vi "20150719_Online_Program_emergency.vi"() -> ()   [LabVIEW 2014]
uses:
  <vilib>/Utility/file.llb/Read From Spreadsheet File (DBL).vi
  <vilib>/Analysis/Matrix/Numeric/Conversions/Array To Matrix - RA2.vi
  <vilib>/Analysis/Matrix/Numeric/Conversions/Array To Matrix - RA.vi
  <vilib>/Utility/file.llb/Write To Spreadsheet File (DBL).vi
  <vilib>/Utility/file.llb/Write To Spreadsheet File (I64).vi
  <vilib>/Analysis/Matrix/NI_Matrix.lvlib
  <vilib>/Instr/_visa.llb/VISA Configure Serial Port (Instr).vi
  NeuroSky_Dll_Call/Debug/NeuroSky_Dll_Call.dll
  user32.dll
panel:
  out "에러 출력":errorcluster
  out "메시지 2":string
  out "큐사인":bool
  out "icon_온도":bool
  out "icon_용변":bool
  out "icon_자판":bool
  out "icon_응급":bool=TRUE
  out "icon_기계":bool
  out "icon_침대":bool
  out "메시지":string
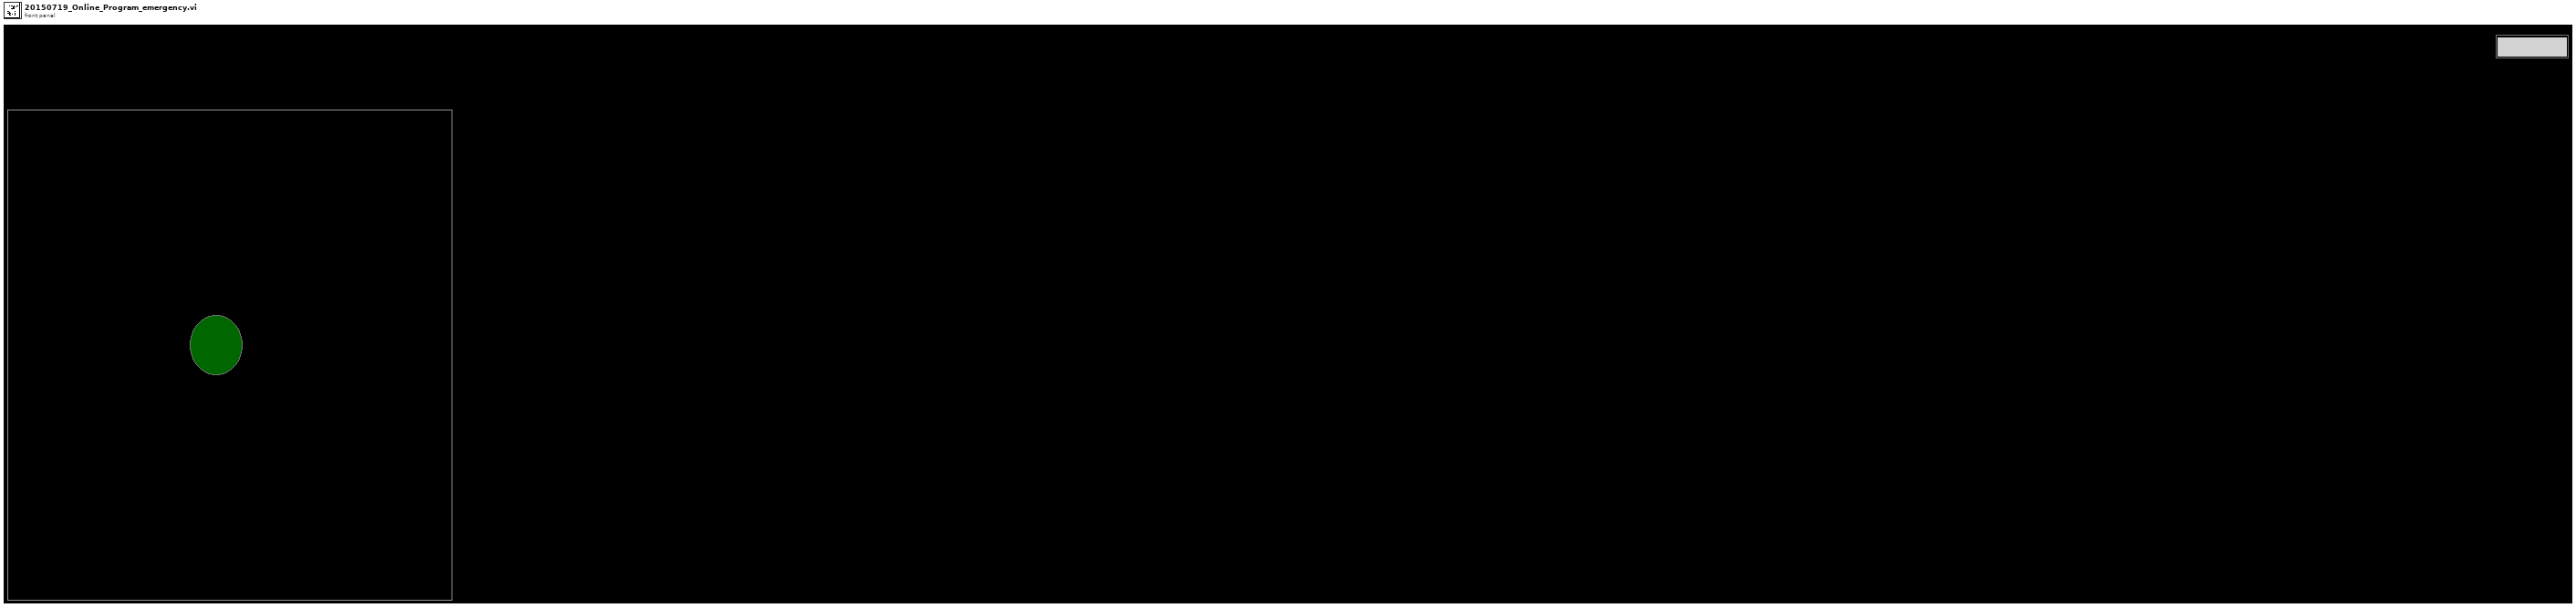
[diagram p1: front panel]
types:
  T1 = typedef "NI_Matrix.lvlib/RealMatrix.ctl" = dbl[][]
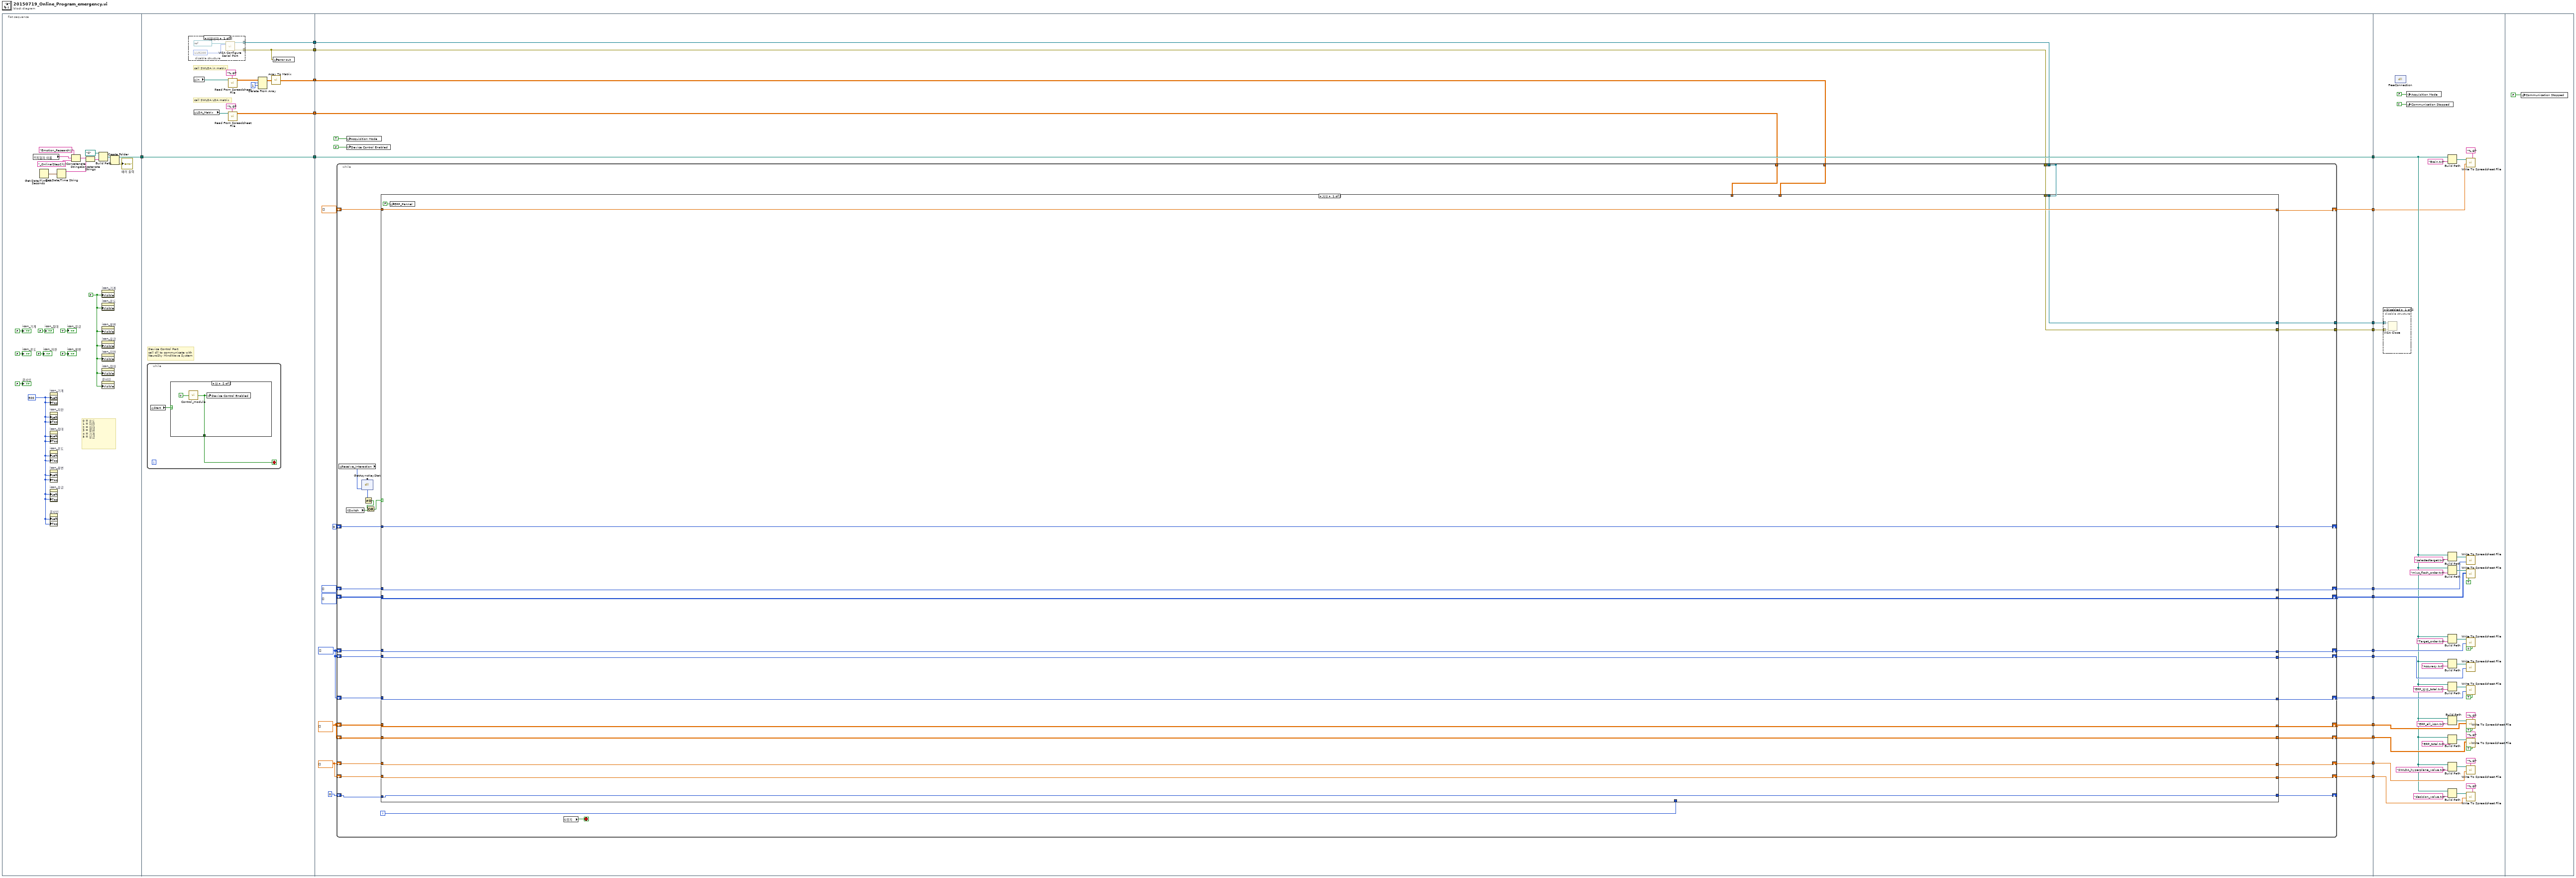
[diagram p0: block diagram]
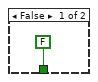
[diagram p3: hidden frame]
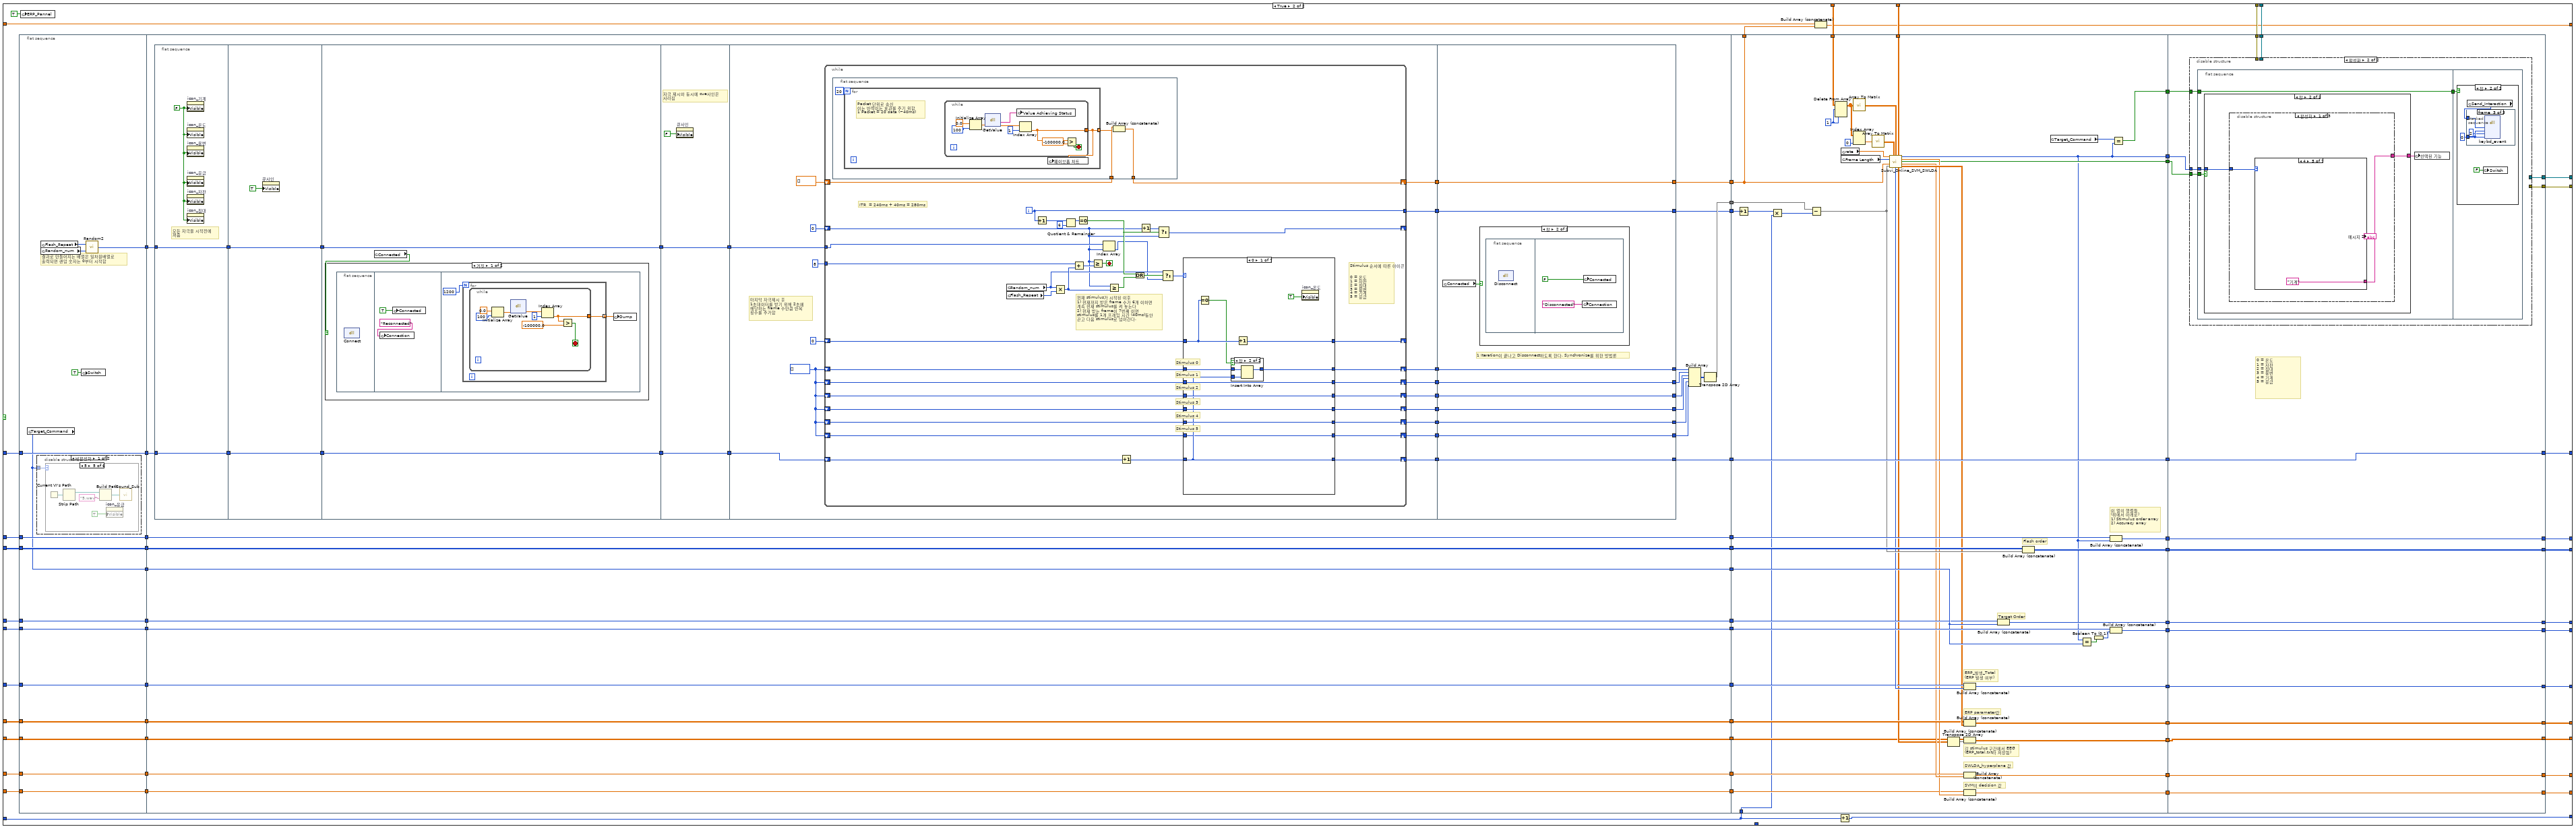
[diagram p4: hidden frame]
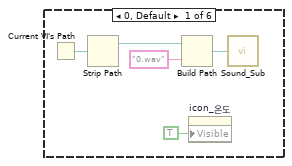
[diagram p5: hidden frame]
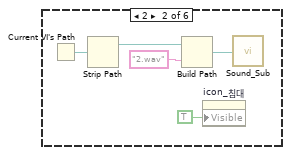
[diagram p6: hidden frame]
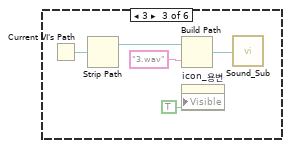
[diagram p7: hidden frame]
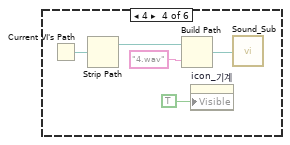
[diagram p8: hidden frame]
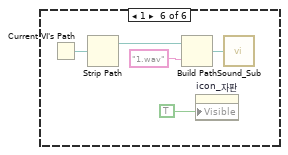
[diagram p9: hidden frame]
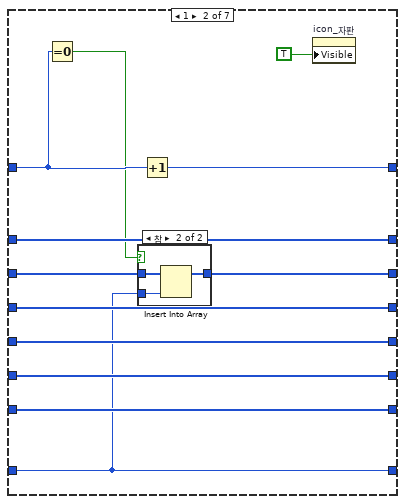
[diagram p13: hidden frame]
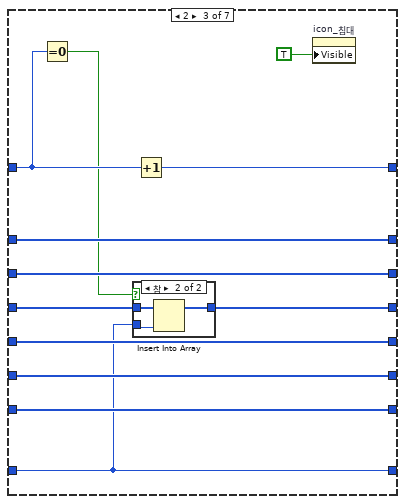
[diagram p15: hidden frame]
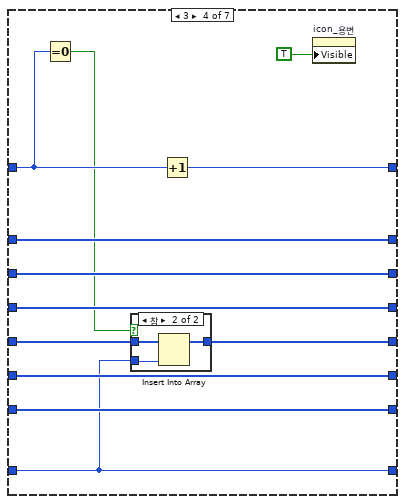
[diagram p17: hidden frame]
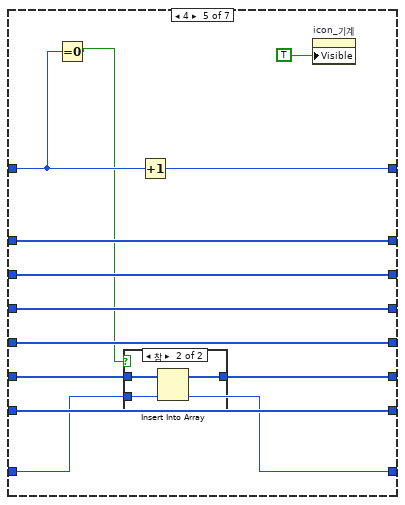
[diagram p19: hidden frame]
diagram:
  n1 = flat-sequence {
    tunnel: [w39] -> w19
    tunnel: w19 -> [w51]
    tunnel: [w51] -> w18
    tunnel: [w49] -> w17
    tunnel: [w42] -> w7
    tunnel: [w41] -> w4
    tunnel: [w40] -> w3
    tunnel: w18 -> [w78]
    tunnel: [w78] -> w16
    tunnel: [w87] -> w15
    tunnel: [w85] -> w14
    tunnel: [w83] -> w13
    tunnel: w17 -> [w68]
    tunnel: [w82] -> w12
    tunnel: [w79] -> w11
    tunnel: [w75] -> w10
    tunnel: [w74] -> w9
    tunnel: [w73] -> w8
    tunnel: w7 -> [w67]
    tunnel: [w71] -> w6
    tunnel: [w69] -> w5
    tunnel: w4 -> [w66]
    tunnel: w3 -> [w65]
    tunnel: [w64] -> w2
    tunnel: [w63] -> w1
    tunnel: w16 -> [w725]
    tunnel: w15 -> [w720]
    tunnel: w14 -> [w759]
    tunnel: w13 -> [w755]
    tunnel: w12 -> [w752]
    tunnel: w11 -> [w748]
    tunnel: w10 -> [w742]
    tunnel: w9 -> [w737]
    tunnel: w8 -> [w734]
    tunnel: w6 -> [w731]
    tunnel: w5 -> [w726]
    tunnel: w2 -> [w722]
    tunnel: w1 -> [w721]
    frame #0 {
      w21 = FALSE ("Visible")
      w22 = 500 ("Position:Left")
      # "0 = 온도\n1 = 자판\n2 = 침대\n3 = 용변 \n4 = 기계 \n5 = 응급"
      n2 = global read "Control_Panel_정리.vi" "피험자 이름"() -> (w30:string)
      n3 = Get Date/Time In Seconds() -> (seconds since 1Jan1904=w36:timestamp)
      n4 = property on="icon_기계" class="Bool (엄격한)"("Left"=w22, "Top"=w22) -> ()  [unwired: 2 in, 2 out]
      n5 = property on="icon_자판" class="Bool (엄격한)"("Left"=w22, "Top"=w22) -> ()  [unwired: 2 in, 2 out]
      n6 = property on="icon_침대" class="Bool (엄격한)"("Left"=w22, "Top"=w22) -> ()  [unwired: 2 in, 2 out]
      n7 = property on="icon_온도" class="Bool (엄격한)"("Left"=w22, "Top"=w22) -> ()  [unwired: 2 in, 2 out]
      n8 = property on="icon_용변" class="Bool (엄격한)"("Left"=w22, "Top"=w22) -> ()  [unwired: 2 in, 2 out]
      n9 = property on="icon_응급" class="Bool (엄격한)"("Left"=w22, "Top"=w22) -> ()  [unwired: 2 in, 2 out]
      n10 = property on="큐사인" class="Bool (엄격한)"("Left"=w22, "Top"=w22) -> ()  [unwired: 2 in, 2 out]
      n11 = Get Date/Time String(seconds (now)=w36) -> (date string=w37:string)  [unwired: 2 in, 1 out]
      n12 = Concatenate Strings("Emotion_Research\\" ("string"), w30, "_Online(Step2)\\" ("문자열")) -> (w32:string)
      n13 = Concatenate Strings(w32, w37) -> (w34:string)
      n14 = Build Path(base path=path "C:/" ("path"), name or relative path=w34) -> (appended path=w35:path)
      n15 = property on="icon_기계" class="Bool (엄격한)"("Visible"=w21) -> ()  [unwired: 2 in, 2 out]
      n16 = property on="icon_온도" class="Bool (엄격한)"("Visible"=w21) -> ()  [unwired: 2 in, 2 out]
      n17 = property on="icon_용변" class="Bool (엄격한)"("Visible"=w21) -> ()  [unwired: 2 in, 2 out]
      n18 = property on="icon_응급" class="Bool (엄격한)"("Visible"=w21) -> ()  [unwired: 2 in, 2 out]
      n19 = property on="icon_자판" class="Bool (엄격한)"("Visible"=w21) -> ()  [unwired: 2 in, 2 out]
      n20 = property on="icon_침대" class="Bool (엄격한)"("Visible"=w21) -> ()  [unwired: 2 in, 2 out]
      n21 = property on="큐사인" class="Bool (엄격한)"("Visible"=w21) -> ()  [unwired: 2 in, 2 out]
      n22 = Create Folder(path (use dialog)=w35) -> (created path=w39:path, error out=→"에러 출력":errorcluster)  [unwired: 2 in, 1 out]
      "icon_온도" <- FALSE ("icon_전원 6")
      "icon_용변" <- FALSE ("icon_전체종료")
      "icon_자판" <- FALSE ("icon_음량업 2")
      "icon_응급" <- TRUE ("icon_채널다운")
      "icon_기계" <- FALSE ("icon_음량다")
      "icon_침대" <- FALSE ("icon_채널업")
      "큐사인" <- FALSE ("icon_전원 7")
    }
    frame #1 {
      w45 = 1 ("인덱스 (행)")
      # "call SWLDA in matrix"
      # "call SWLDA LDA matrix"
      # "Device Control Part\ncall dll to communicate with\nNeuroSky MindWave System"
      n23 = while {
        stop <- w57 stop-if-true
        n24 = global read "Control_Panel_정리.vi" "Start"() -> (w56:bool)
        n25 = case shown="참" w56 {
          tunnel: [FALSE ("Connected") w59] -> w57
          frame False {
          }
          frame True {
            n26 = call "Control_module.vi"("Turn on"=TRUE ("Device Control Enabled")) -> ("Connected"=w59:bool)
            n27 = global write "Control_Panel_정리.vi" "Device Control Enabled"(w59) -> ()
          }
        }
      }
      n28 = disable-structure shown="비활성화" {
        disable-tunnel: [w55 _] -> w41
        disable-tunnel: [w54 _] -> w40
        frame Disabled {
          n29 = call-poly "VISA Configure Serial Port"("VISA resource name"=refnum<visa-resource-name> "COM3", "baud rate (9600)"=u32 115200) -> ("VISA resource name out"=w55:refnum<visa-resource-name>, "error out"=w54:errorcluster)  [unwired: 12 in]
        }
        frame Enabled {
        }
      }
      n30 = global read "Control_Panel_정리.vi" "in"() -> (w43:path)
      n31 = global read "Control_Panel_정리.vi" "LDA_Matrix"() -> (w48:path)
      n32 = call-poly <vilib>:"Read From Spreadsheet File.vi"("format (%.3f)"="%.6f", "file path (dialog if empty)"=w43) -> ("all rows"=w44:dbl[][])  [unwired: 5 in, 4 out]
      n33 = call-poly <vilib>:"Read From Spreadsheet File.vi"("format (%.3f)"="%.6f", "file path (dialog if empty)"=w48) -> ("all rows"=w49:dbl[][])  [unwired: 5 in, 4 out]
      n34 = Delete From Array(array=w44, length=w45, index (row)=w45) -> (array with subset deleted=w46:dbl[][])  [unwired: 1 in, 1 out]
      n35 = call-poly <vilib>:"Array To Matrix.vi"("Real 2D Array"=w46) -> ("Real Matrix"=w42:T1)
      n36 = global write "Control_Panel_정리.vi" "error out"(w40) -> ()
    }
    frame #2 {
      w72 = dbl[] []
      w70 = dbl[][] []
      w62 = i16[] []
      n37 = while {
        shift-right: [w96] -> w87
        shift-left: dbl[] [] -> [w102]
        shift-right: [w123] -> _
        shift-left: 0 ("y") -> [w124]
        shift-right: [w117] -> w85
        shift-left: i32[][] [] -> [w118]
        shift-right: [w121] -> w83
        shift-left: i32[] [] -> [w122]
        shift-right: [w119] -> w82
        shift-left: w62 -> [w120]
        shift-right: [w114] -> w79
        shift-left: w62 -> [w115]
        shift-right: [w113] -> w75
        shift-left: w62 -> [w112]
        shift-right: [w111] -> w74
        shift-left: w70 -> [w110]
        shift-right: [w109] -> w73
        shift-left: w72 -> [w108]
        shift-right: [w107] -> w71
        shift-left: w72 -> [w106]
        shift-right: [w105] -> w69
        shift-left: w70 -> [w104]
        tunnel: w68 -> [w103]
        tunnel: w67 -> [w101]
        tunnel: [w99] -> _
        tunnel: w66 -> [w99]
        tunnel: w65 -> [w100]
        tunnel: [w98] -> w64
        tunnel: [w97] -> w63
        shift-right: [w88] -> _
        shift-left: 0 -> [w89]
        i -> [w116]
        stop <- w95 stop-if-true
        n38 = global read "Control_Panel_정리.vi" "Receive_Interaction"() -> (w93:u8)
        n39 = global read "Control_Panel_정리.vi" "Switch"() -> (w91:bool)
        n40 = dll-call lib="User32.dll" fn="GetAsyncKeyState"("vKey"=w93) -> ("return type"=w94:i64)  [unwired: 4 in, 2 out]
        n41 = Not Equal To 0?(x=w94) -> (x != 0?=w92:bool)
        n42 = Or(x=w92, y=w91) -> (x .or. y?=w90:bool)
        n43 = case shown="거짓" w90 {
          tunnel: w124 -> [w136 w173]
          tunnel: [w136 w172] -> w123
          tunnel: w122 -> [w135 w171]
          tunnel: [w135 w170] -> w121
          tunnel: w120 -> [w132 w169]
          tunnel: [w132 w168] -> w119
          tunnel: w118 -> [w134 w167]
          tunnel: [w134 w166] -> w117
          tunnel: w116 -> [_ _]
          tunnel: w115 -> [w133 w165]
          tunnel: [w133 w164] -> w114
          tunnel: [w131 w163] -> w113
          tunnel: w112 -> [w131 w162]
          tunnel: [w130 w161] -> w111
          tunnel: w110 -> [w130 w160]
          tunnel: [w128 w159] -> w109
          tunnel: w108 -> [w128 w158]
          tunnel: [w127 w157] -> w107
          tunnel: w106 -> [w127 w156]
          tunnel: [w129 w155] -> w105
          tunnel: w104 -> [w129 w154]
          tunnel: w103 -> [_ w153]
          tunnel: w102 -> [w139 w152]
          tunnel: w101 -> [_ w150]
          tunnel: w100 -> [w137 w149]
          tunnel: w99 -> [w138 w148]
          tunnel: [w138 w147] -> w98
          tunnel: [w137 w146] -> w97
          tunnel: [w139 w145] -> w96
          tunnel: w89 -> [w125 w141]
          tunnel: [w125 w140] -> w88
          frame False {
            n44 = global write "Control_Panel_정리.vi" "ERP_Pannel"(FALSE ("ERP_Pannel")) -> ()
          }
          frame True {
            n45 = flat-sequence {
              tunnel: w173 -> [w225]
              tunnel: [w225] -> w210
              tunnel: [w215] -> w209
              tunnel: w171 -> [w224]
              tunnel: [w224] -> w208
              tunnel: w169 -> [w223]
              tunnel: [w223] -> w207
              tunnel: w167 -> [w222]
              tunnel: [w222] -> w206
              tunnel: [w221] -> w205
              tunnel: w165 -> [w221]
              tunnel: w162 -> [w220]
              tunnel: [w220] -> w204
              tunnel: w160 -> [w219]
              tunnel: [w219] -> w203
              tunnel: w158 -> [w218]
              tunnel: [w218] -> w202
              tunnel: w156 -> [w217]
              tunnel: [w217] -> w201
              tunnel: w154 -> [w216]
              tunnel: [w216] -> w200
              tunnel: [w211] -> w142
              tunnel: w210 -> [w294]
              tunnel: [w295] -> w199
              tunnel: [w284] -> w198
              tunnel: [w293] -> w197
              tunnel: [w292] -> w196
              tunnel: w209 -> [w291]
              tunnel: [w291] -> w195
              tunnel: w208 -> [w290]
              tunnel: [w290] -> w194
              tunnel: [w289] -> w193
              tunnel: w207 -> [w289]
              tunnel: [w288] -> w192
              tunnel: w206 -> [w288]
              tunnel: [w287] -> w191
              tunnel: w205 -> [w287]
              tunnel: [w286] -> w190
              tunnel: w204 -> [w286]
              tunnel: [w285] -> w189
              tunnel: w203 -> [w285]
              tunnel: [w283] -> w188
              tunnel: w202 -> [w283]
              tunnel: [w282] -> w187
              tunnel: w201 -> [w282]
              tunnel: w200 -> [w281]
              tunnel: [w281] -> w186
              tunnel: w142 -> [w260]
              tunnel: w199 -> [w539]
              tunnel: w198 -> [w513]
              tunnel: w197 -> [w551]
              tunnel: w196 -> [w552]
              tunnel: [w551] -> w175
              tunnel: [w511] -> w176
              tunnel: w195 -> [w538]
              tunnel: w194 -> [w547]
              tunnel: [w546] -> w177
              tunnel: w193 -> [w544]
              tunnel: [w543] -> w178
              tunnel: w192 -> [w542]
              tunnel: [w540] -> w179
              tunnel: w191 -> [w537]
              tunnel: [w536] -> w180
              tunnel: [w534] -> w181
              tunnel: w190 -> [w533]
              tunnel: [w531] -> w182
              tunnel: w189 -> [w530]
              tunnel: [w528] -> w183
              tunnel: w188 -> [w527]
              tunnel: [w525] -> w184
              tunnel: w187 -> [w524]
              tunnel: [w521] -> w185
              tunnel: w186 -> [w520]
              tunnel: w153 -> [w519]
              tunnel: [w513] -> w151
              tunnel: w150 -> [w515]
              tunnel: [w514] -> w174
              tunnel: [w510] -> w144
              tunnel: w141 -> [w509]
              tunnel: [w574] -> w172
              tunnel: [w573] -> w170
              tunnel: [w570] -> w168
              tunnel: [w572] -> w166
              tunnel: [w571] -> w164
              tunnel: [w569] -> w163
              tunnel: [w568] -> w161
              tunnel: [w567] -> w159
              tunnel: [w566] -> w157
              tunnel: [w565] -> w155
              tunnel: w185 -> [w565]
              tunnel: w184 -> [w566]
              tunnel: w183 -> [w567]
              tunnel: w182 -> [w568]
              tunnel: w181 -> [w569]
              tunnel: w180 -> [w571]
              tunnel: w179 -> [w572]
              tunnel: w178 -> [w570]
              tunnel: w177 -> [w573]
              tunnel: w176 -> [w564]
              tunnel: w175 -> [w574]
              tunnel: w174 -> [w563]
              tunnel: w149 -> [w562]
              tunnel: w148 -> [w561]
              tunnel: [w560] -> w147
              tunnel: [w559] -> w146
              tunnel: w144 -> [w558]
              frame #0 {
                # "결과로 만들어지는 배열은 일차원배열로\n출력되면 랜덤 숫자는 0부터 시작함"
                n46 = global read "Control_Panel_정리.vi" "Target_Command"() -> (w215:i32)
                n47 = disable-structure shown="비활성화" {
                  disable-tunnel: w215 -> [w226 _]
                  frame Disabled {
                    n48 = case shown="5" w226 {
                      frame 0, Default {
                        n49 = Current VI's Path() -> (path=w229:path)
                        n50 = Strip Path(path=w229) -> (stripped path=w230:path)  [unwired: 1 out]
                        n51 = Build Path(base path=w230, name or relative path="0.wav" ("이름 또는 상대 경로")) -> (appended path=w228:path)
                        n52 = property on="icon_온도" class="Bool (엄격한)"("Visible"=TRUE) -> ()  [unwired: 2 in, 2 out]
                        n53 = call "Sound_Sub.vi"("path"=w228) -> ()
                      }
                      frame 2 {
                        n54 = Current VI's Path() -> (path=w233:path)
                        n55 = Strip Path(path=w233) -> (stripped path=w234:path)  [unwired: 1 out]
                        n56 = Build Path(base path=w234, name or relative path="2.wav" ("이름 또는 상대 경로")) -> (appended path=w236:path)
                        n57 = property on="icon_침대" class="Bool (엄격한)"("Visible"=TRUE) -> ()  [unwired: 2 in, 2 out]
                        n58 = call "Sound_Sub.vi"("path"=w236) -> ()
                      }
                      frame 3 {
                        n59 = Current VI's Path() -> (path=w238:path)
                        n60 = Strip Path(path=w238) -> (stripped path=w239:path)  [unwired: 1 out]
                        n61 = Build Path(base path=w239, name or relative path="3.wav" ("이름 또는 상대 경로")) -> (appended path=w241:path)
                        n62 = property on="icon_용변" class="Bool (엄격한)"("Visible"=TRUE) -> ()  [unwired: 2 in, 2 out]
                        n63 = call "Sound_Sub.vi"("path"=w241) -> ()
                      }
                      frame 4 {
                        n64 = Current VI's Path() -> (path=w243:path)
                        n65 = Strip Path(path=w243) -> (stripped path=w244:path)  [unwired: 1 out]
                        n66 = Build Path(base path=w244, name or relative path="4.wav" ("이름 또는 상대 경로")) -> (appended path=w246:path)
                        n67 = property on="icon_기계" class="Bool (엄격한)"("Visible"=TRUE) -> ()  [unwired: 2 in, 2 out]
                        n68 = call "Sound_Sub.vi"("path"=w246) -> ()
                      }
                      frame 5 {
                        n69 = Current VI's Path() -> (path=w248:path)
                        n70 = Strip Path(path=w248) -> (stripped path=w249:path)  [unwired: 1 out]
                        n71 = Build Path(base path=w249, name or relative path="5.wav" ("이름 또는 상대 경로")) -> (appended path=w251:path)
                        n72 = property on="icon_응급" class="Bool (엄격한)"("Visible"=TRUE) -> ()  [unwired: 2 in, 2 out]
                        n73 = call "Sound_Sub.vi"("path"=w251) -> ()
                      }
                      frame 1 {
                        n74 = Current VI's Path() -> (path=w254:path)
                        n75 = Strip Path(path=w254) -> (stripped path=w255:path)  [unwired: 1 out]
                        n76 = Build Path(base path=w255, name or relative path="1.wav" ("이름 또는 상대 경로")) -> (appended path=w253:path)
                        n77 = property on="icon_자판" class="Bool (엄격한)"("Visible"=TRUE) -> ()  [unwired: 2 in, 2 out]
                        n78 = call "Sound_Sub.vi"("path"=w253) -> ()
                      }
                    }
                  }
                  frame Enabled {
                  }
                }
                n79 = global read "Control_Panel_정리.vi" "Flash_Repeat"() -> (w212:i32)
                n80 = global read "Control_Panel_정리.vi" "Random_num"() -> (w213:i32)
                n81 = global write "Control_Panel_정리.vi" "Switch"(TRUE ("Switch")) -> ()
                n82 = call "Random2.vi"("Random_num"=w213, "전체횟수"=w212) -> ("배열"=w211:i32[])
              }
              frame #1 {
                n83 = flat-sequence {
                  tunnel: w294 -> [w299]
                  tunnel: [w299] -> w280
                  tunnel: [w297] -> w261
                  tunnel: w260 -> [w297]
                  tunnel: [w302] -> w273
                  tunnel: w280 -> [w302]
                  tunnel: w261 -> [w300]
                  tunnel: [w300] -> w257
                  tunnel: w273 -> [w305]
                  tunnel: [w305] -> w263
                  tunnel: [w303] -> w258
                  tunnel: w257 -> [w303]
                  tunnel: w263 -> [w321]
                  tunnel: [w321] -> w262
                  tunnel: [w319] -> w259
                  tunnel: w258 -> [w319]
                  tunnel: w262 -> [w328]
                  tunnel: [w336] -> w272
                  tunnel: [w335] -> w271
                  tunnel: [w334] -> w270
                  tunnel: [w333] -> w269
                  tunnel: [w332] -> w268
                  tunnel: [w327] -> w267
                  tunnel: [w326] -> w266
                  tunnel: [w325] -> w265
                  tunnel: [w323] -> w264
                  tunnel: w259 -> [w322]
                  tunnel: [w498] -> w284
                  tunnel: [w499] -> w276
                  tunnel: [w500] -> w292
                  tunnel: [w501] -> w293
                  tunnel: [w502] -> w279
                  tunnel: [w503] -> w278
                  tunnel: [w504] -> w277
                  tunnel: [w505] -> w275
                  tunnel: [w506] -> w274
                  tunnel: w272 -> [w506]
                  tunnel: w271 -> [w505]
                  tunnel: w270 -> [w504]
                  tunnel: w269 -> [w503]
                  tunnel: w268 -> [w502]
                  tunnel: w267 -> [w501]
                  tunnel: w266 -> [w500]
                  tunnel: w265 -> [w499]
                  tunnel: w264 -> [w498]
                  frame #0 {
                    w298 = FALSE ("Visible")
                    # "모든 자극을 시작전에\n꺼줌"
                    n84 = property on="icon_기계" class="Bool (엄격한)"("Visible"=w298) -> ()  [unwired: 2 in, 2 out]
                    n85 = property on="icon_온도" class="Bool (엄격한)"("Visible"=w298) -> ()  [unwired: 2 in, 2 out]
                    n86 = property on="icon_용변" class="Bool (엄격한)"("Visible"=w298) -> ()  [unwired: 2 in, 2 out]
                    n87 = property on="icon_응급" class="Bool (엄격한)"("Visible"=w298) -> ()  [unwired: 2 in, 2 out]
                    n88 = property on="icon_자판" class="Bool (엄격한)"("Visible"=w298) -> ()  [unwired: 2 in, 2 out]
                    n89 = property on="icon_침대" class="Bool (엄격한)"("Visible"=w298) -> ()  [unwired: 2 in, 2 out]
                  }
                  frame #1 {
                    n90 = property on="큐사인" class="Bool (엄격한)"("Visible"=TRUE) -> ()  [unwired: 2 in, 2 out]
                  }
                  frame #2 {
                    n91 = global read "Control_Panel_정리.vi" "Connected"() -> (w304:bool)
                    n92 = case shown="거짓" w304 {
                      frame False {
                        n93 = flat-sequence {
                          frame #0 {
                            n94 = dll-call lib="C:/Users/Server/Desktop/NeuroSky/NeuroSky_Dll_Call/Debug/NeuroSky_Dll_Call.dll" fn="Connect"() -> ()  [unwired: 4 in, 2 out]
                          }
                          frame #1 {
                            n95 = global write "Control_Panel_정리.vi" "Connection"("Reconnected") -> ()
                            n96 = global write "Control_Panel_정리.vi" "Connected"(TRUE ("Connected")) -> ()
                          }
                          frame #2 {
                            n97 = for {
                              N: 1200 -> [_]
                              tunnel: [w310] -> w308 mode=indexing
                              n98 = while {
                                tunnel: [w312] -> w310
                                stop <- w311 stop-if-true
                                n99 = Initialize Array(0.0 ("element"), 100 ("dimension size")) -> (w317:dbl[])
                                n100 = dll-call lib="C:/Users/Server/Desktop/NeuroSky/NeuroSky_Dll_Call/Debug/NeuroSky_Dll_Call.dll" fn="GetValue"("result"=w317) -> ("result"=w318:dbl[])  [unwired: 4 in, 2 out]
                                n101 = Index Array(array=w318, index=1) -> (element=w312:dbl)
                                n102 = Greater?(x=w312, y=-100000.0) -> (0:w311:bool)
                              }
                            }
                            n103 = global write "Control_Panel_정리.vi" "Dump"(w308) -> ()
                          }
                        }
                      }
                      frame True {
                      }
                    }
                  }
                  frame #3 {
                    # "자극 제시와 동시에 cue사인은\n사라짐"
                    n104 = property on="큐사인" class="Bool (엄격한)"("Visible"=FALSE) -> ()  [unwired: 2 in, 2 out]
                  }
                  frame #4 {
                    w330 = i32[] []
                    # "마지막 자극제시 후\n1초데이터를 받기 위해 2초에\n해당하는 frame 수만큼 반복\n횟수를 추가함"
                    n105 = while {
                      shift-right: [w344] -> w323
                      shift-left: dbl[] [] -> [w345]
                      tunnel: 8 -> [w341]
                      shift-right: [w371] -> w336
                      shift-left: w330 -> [w370]
                      shift-right: [w368] -> w335
                      shift-left: w330 -> [w369]
                      shift-right: [w366] -> w325
                      shift-left: w330 -> [w367]
                      shift-right: [w364] -> w334
                      shift-left: w330 -> [w365]
                      shift-right: [w362] -> w333
                      shift-left: w330 -> [w363]
                      shift-right: [w361] -> w332
                      shift-left: w330 -> [w349]
                      shift-right: [w359] -> w327
                      shift-left: w328 -> [w360]
                      shift-right: [w355] -> _
                      shift-left: 0 -> [w339]
                      shift-right: [w350] -> _
                      shift-left: 0 ("y") -> [w351]
                      tunnel: [w346] -> w326
                      tunnel: w322 -> [w340]
                      i -> [w346]
                      stop <- w374 stop-if-true
                      # "ITR  = 240ms + 40ms = 280ms"
                      # "현재 stimulus가 시작된 이후\n1) 현재까지 받은 frame 수가 6개 이하면\n계속 현재 stimulus를 켜 놓는다\n2) 현재 받는 frame이 7번째 이면\nstimulus를 1개 프레임 시간 (40ms)동안\n끈고 다음 stimulus로 넘어간다."
                      # "Stimulus 순서에 따른 아이콘\n\n\n0 = 온도\n1 = 자판\n2 = 침대\n3 = 용변 \n4 = 기계 \n5 = 응급"
                      # "Stimulus 5"
                      # "Stimulus 4"
                      # "Stimulus 3"
                      # "Stimulus 2"
                      # "Stimulus 1"
                      # "Stimulus 0"
                      n106 = flat-sequence {
                        tunnel: [w379] -> w344
                        tunnel: w345 -> [w378]
                        frame #0 {
                          n107 = for {
                            N: 20 -> [_]
                            tunnel: [w380] -> w377 mode=indexing
                            # "Packet 단위로 송신\n이는 반짝이는 효과를 주기 위함\n1 Packet = 20 data (~40ms)"
                            n108 = while {
                              tunnel: [w382] -> w380
                              stop <- w381 stop-if-true
                              n109 = Initialize Array(0.0 ("element"), 100 ("dimension size")) -> (w388:dbl[])
                              n110 = dll-call lib="C:/Users/Server/Desktop/NeuroSky/NeuroSky_Dll_Call/Debug/NeuroSky_Dll_Call.dll" fn="GetValue"("result"=w388) -> ("errCode"=w384:string, "result"=w389:dbl[])  [unwired: 3 in, 2 out]
                              n111 = global write "Control_Panel_정리.vi" "Value Achieving Status"(w384) -> ()
                              n112 = Index Array(array=w389, index=1) -> (element=w382:dbl)
                              n113 = Greater?(x=w382, y=-100000.0) -> (0:w381:bool)
                            }
                            n114 = global write "Control_Panel_정리.vi" "웨이브폼 차트"(w380) -> ()
                          }
                          n115 = Build Array (concatenate)(w378, w377) -> (w379:dbl[])
                        }
                      }
                      n116 = global read "Control_Panel_정리.vi" "Random_num"() -> (w343:i32)
                      n117 = global read "Control_Panel_정리.vi" "Flash_Repeat"() -> (w342:i32)
                      n118 = Increment(x=w346) -> (x+1=w348:i32)
                      n119 = Multiply(x=w343, y=w342) -> (x*y=w347:i32)
                      n120 = Quotient & Remainder(x=w348, y=6) -> (x-y*floor(x/y)=w357:i32)  [unwired: 1 out]
                      n121 = Add(x=w341, y=w347) -> (x+y=w375:i32)
                      n122 = Equal To 0?(x=w357) -> (x = 0?=w354:bool)
                      n123 = Greater Or Equal?(x=w339, y=w375) -> (x >= y?=w374:bool)
                      n124 = Index Array(array=w340, index=w339) -> (element=w338:i32)
                      n125 = Greater Or Equal?(x=w339, y=w347) -> (x >= y?=w353:bool)
                      n126 = Increment(x=w360) -> (x+1=w372:i32)
                      n127 = Or(x=w354, y=w353) -> (x .or. y?=w352:bool)
                      n128 = Increment(x=w339) -> (x+1=w356:i32)
                      n129 = Select(t=w356, s=w354, f=w339) -> (s? t:f=w355:i32)
                      n130 = Select(t=w343, s=w352, f=w338) -> (s? t:f=w373:i32)
                      n131 = case shown="0" w373 {
                        tunnel: w372 -> [w395 w411 w426 w442 w458 w475 w490]
                        tunnel: [w400 w408 w433 w449 w465 w481 w496] -> w371
                        tunnel: w370 -> [w401 w408 w433 w449 w465 w481 w496]
                        tunnel: w369 -> [w399 w417 w430 w446 w462 w479 w495]
                        tunnel: [w399 w416 w430 w446 w462 w479 w495] -> w368
                        tunnel: w367 -> [w398 w415 w432 w445 w461 w478 w494]
                        tunnel: [w398 w415 w431 w445 w461 w478 w494] -> w366
                        tunnel: w365 -> [w397 w414 w429 w448 w460 w477 w493]
                        tunnel: [w397 w414 w429 w447 w460 w477 w493] -> w364
                        tunnel: w363 -> [w396 w413 w428 w444 w464 w476 w492]
                        tunnel: [w396 w413 w428 w444 w463 w476 w492] -> w362
                        tunnel: w349 -> [w392 w412 w427 w443 w459 w480 w491]
                        tunnel: [w392 w412 w427 w443 w459 w472 w491] -> w361
                        tunnel: [w395 w411 w426 w442 w458 w475 w490] -> w359
                        tunnel: w351 -> [w394 w410 w425 w440 w457 w473 _]
                        tunnel: [w393 w409 w424 w441 w456 w474 0] -> w350
                        frame 0 {
                          n132 = Equal To 0?(x=w394) -> (x = 0?=w390:bool)
                          n133 = case shown="참" w390 {
                            tunnel: w401 -> [w402 w405]
                            tunnel: [w402 w404] -> w400
                            tunnel: w395 -> [_ w403]
                            frame False {
                            }
                            frame True {
                              n134 = Insert Into Array(array=w405, new element=w403) -> (w404:i32[])  [unwired: 1 in]
                            }
                          }
                          n135 = Increment(x=w394) -> (x+1=w393:i32)
                          n136 = property on="icon_온도" class="Bool (엄격한)"("Visible"=TRUE) -> ()  [unwired: 2 in, 2 out]
                        }
                        frame 1 {
                          n137 = Equal To 0?(x=w410) -> (x = 0?=w406:bool)
                          n138 = case shown="참" w406 {
                            tunnel: w417 -> [w418 w421]
                            tunnel: [w418 w420] -> w416
                            tunnel: w411 -> [_ w419]
                            frame False {
                            }
                            frame True {
                              n139 = Insert Into Array(array=w421, new element=w419) -> (w420:i32[])  [unwired: 1 in]
                            }
                          }
                          n140 = Increment(x=w410) -> (x+1=w409:i32)
                          n141 = property on="icon_자판" class="Bool (엄격한)"("Visible"=TRUE) -> ()  [unwired: 2 in, 2 out]
                        }
                        frame 2 {
                          n142 = Equal To 0?(x=w425) -> (x = 0?=w422:bool)
                          n143 = case shown="참" w422 {
                            tunnel: w432 -> [w434 w437]
                            tunnel: [w434 w436] -> w431
                            tunnel: w426 -> [_ w435]
                            frame False {
                            }
                            frame True {
                              n144 = Insert Into Array(array=w437, new element=w435) -> (w436:i32[])  [unwired: 1 in]
                            }
                          }
                          n145 = Increment(x=w425) -> (x+1=w424:i32)
                          n146 = property on="icon_침대" class="Bool (엄격한)"("Visible"=TRUE) -> ()  [unwired: 2 in, 2 out]
                        }
                        frame 3 {
                          n147 = Equal To 0?(x=w440) -> (x = 0?=w438:bool)
                          n148 = case shown="참" w438 {
                            tunnel: w448 -> [w450 w453]
                            tunnel: [w450 w452] -> w447
                            tunnel: w442 -> [_ w451]
                            frame False {
                            }
                            frame True {
                              n149 = Insert Into Array(array=w453, new element=w451) -> (w452:i32[])  [unwired: 1 in]
                            }
                          }
                          n150 = Increment(x=w440) -> (x+1=w441:i32)
                          n151 = property on="icon_용변" class="Bool (엄격한)"("Visible"=TRUE) -> ()  [unwired: 2 in, 2 out]
                        }
                        frame 4 {
                          n152 = Equal To 0?(x=w457) -> (x = 0?=w454:bool)
                          n153 = case shown="참" w454 {
                            tunnel: w464 -> [w466 w469]
                            tunnel: [w466 w468] -> w463
                            tunnel: w458 -> [_ w467]
                            frame False {
                            }
                            frame True {
                              n154 = Insert Into Array(array=w469, new element=w467) -> (w468:i32[])  [unwired: 1 in]
                            }
                          }
                          n155 = Increment(x=w457) -> (x+1=w456:i32)
                          n156 = property on="icon_기계" class="Bool (엄격한)"("Visible"=TRUE) -> ()  [unwired: 2 in, 2 out]
                        }
                        frame 5 {
                          n157 = Equal To 0?(x=w473) -> (x = 0?=w470:bool)
                          n158 = case shown="참" w470 {
                            tunnel: w480 -> [w482 w485]
                            tunnel: [w482 w484] -> w472
                            tunnel: w475 -> [_ w483]
                            frame False {
                            }
                            frame True {
                              n159 = Insert Into Array(array=w485, new element=w483) -> (w484:i32[])  [unwired: 1 in]
                            }
                          }
                          n160 = Increment(x=w473) -> (x+1=w474:i32)
                          n161 = property on="icon_응급" class="Bool (엄격한)"("Visible"=TRUE) -> ()  [unwired: 2 in, 2 out]
                        }
                        frame 6, Default {
                          w487 = FALSE ("Visible")
                          w488 = FALSE ("Visible")
                          w486 = FALSE ("Visible")
                          n162 = property on="icon_기계" class="Bool (엄격한)"("Visible"=w486) -> ()  [unwired: 2 in, 2 out]
                          n163 = property on="icon_온도" class="Bool (엄격한)"("Visible"=w486) -> ()  [unwired: 2 in, 2 out]
                          n164 = property on="icon_응급" class="Bool (엄격한)"("Visible"=w488) -> ()  [unwired: 2 in, 2 out]
                          n165 = property on="icon_용변" class="Bool (엄격한)"("Visible"=w488) -> ()  [unwired: 2 in, 2 out]
                          n166 = property on="icon_자판" class="Bool (엄격한)"("Visible"=w487) -> ()  [unwired: 2 in, 2 out]
                          n167 = property on="icon_침대" class="Bool (엄격한)"("Visible"=w487) -> ()  [unwired: 2 in, 2 out]
                        }
                      }
                    }
                  }
                  frame #5 {
                    # "1 Iteration이 끝나고 Disconnect하도록 한다. Synchronize를 위한 방법론"
                    n168 = global read "Control_Panel_정리.vi" "Connected"() -> (w497:bool)
                    n169 = case shown="참" w497 {
                      frame False {
                      }
                      frame True {
                        n170 = flat-sequence {
                          frame #0 {
                            n171 = dll-call lib="C:/Users/Server/Desktop/NeuroSky/NeuroSky_Dll_Call/Debug/NeuroSky_Dll_Call.dll" fn="Disconnect"() -> ()  [unwired: 4 in, 2 out]
                          }
                          frame #1 {
                            n172 = global write "Control_Panel_정리.vi" "Connection"("Disconnected") -> ()
                            n173 = global write "Control_Panel_정리.vi" "Connected"(FALSE ("Connected")) -> ()
                          }
                        }
                      }
                    }
                  }
                }
                n174 = Build Array(w274, w275, w276, w277, w278, w279) -> (w296:i32[][])
                n175 = Transpose 2D Array(2D array=w296) -> (transposed array=w295:i32[][])
              }
              frame #2 {
                w555 = 1 ("인덱스 (행)")
                # "각 stimulus 구간에서 EEG\n(ERP_total.txt라 저장됨)"
                # "ERP parameter값"
                # "SVM의 decision 값"
                # "SWLDA_hyperplane 값"
                # "ERP_발생_Total\n(ERP 발생 여부)"
                # "Target Order"
                # "Flash order"
                # "이 열의 행렬들 \n(위에서 아래로)\n1) Stimulus order array\n2) Accuracy array"
                n176 = Increment(x=w552) -> (x+1=w556:i32)
                n177 = Multiply(x=w556, y=w509) -> (x*y=w557:i32)
                n178 = Subtract(x=w539, y=w557) -> (x-y=w541:i32[][])
                n179 = Delete From Array(array=w519, length=w555, index (row)=w555) -> (array with subset deleted=w517:dbl[][])  [unwired: 1 in, 1 out]
                n180 = global read "Control_Panel_정리.vi" "rate"() -> (w549:dbl)
                n181 = global read "Control_Panel_정리.vi" "Frame Length"() -> (w550:i32)
                n182 = call-poly <vilib>:"Array To Matrix.vi"("Real 2D Array"=w517) -> ("Real Matrix"=w516:T1)
                n183 = Index Array(array=w517, index (col)=0 ("인덱스")) -> (element=w518:dbl[])  [unwired: 1 in]
                n184 = call-poly <vilib>:"Array To Matrix.vi"("Real 1D Array"=w518) -> ("Real Matrix (Column Vector)"=w553:T1)
                n185 = call "Subvi_Online_SVM_SWLDA.vi"("rate"=w549, "Value"=w553, "Matrix"=w516, "in"=w515, "samples per channel"=w550, "Brain_data_source"=w513, "Target_Flash_Order"=w541) -> ("output-0~8"=w511:i32, "decision"=w526:dbl[], "ERP_발생여부"=w514:bool, "SWLDA"=w529:dbl[], "EPR_발생_total"=w535:i16[], "ERP_all"=w523:dbl[][], "ERP_Parameters"=w532:dbl[][])  [unwired: 2 in]
                n186 = Transpose 2D Array(2D array=w523) -> (transposed array=w522:dbl[][])
                n187 = Build Array (concatenate)(w533, w535) -> (w534:i16[])
                n188 = Build Array (concatenate)(w530, w532) -> (w531:dbl[][])
                n189 = Build Array (concatenate)(w520, w522) -> (w521:dbl[][])
                n190 = Build Array (concatenate)(w527, w529) -> (w528:dbl[])
                n191 = Build Array (concatenate)(w524, w526) -> (w525:dbl[])
                n192 = Build Array (concatenate)(w537, w538) -> (w536:i32[])
                n193 = Build Array (concatenate)(w542, w541) -> (w540:i32[][])
                n194 = global read "Control_Panel_정리.vi" "Target_Command"() -> (w512:i32)
                n195 = Equal?(x=w511, y=w538) -> (x = y?=w548:bool)
                n196 = Boolean To (0,1)(Boolean=w548) -> (0, 1=w545:i16)
                n197 = Build Array (concatenate)(w547, w511) -> (w546:i32[])
                n198 = Build Array (concatenate)(w544, w545) -> (w543:i16[])
                n199 = Equal?(x=w512, y=w511) -> (x = y?=w510:bool)
              }
              frame #3 {
                # "0 = 온도\n1 = 자판\n2 = 침대\n3 = 용변 \n4 = 기계 \n5 = 응급"
                n200 = disable-structure shown="활성화" {
                  disable-tunnel: w564 -> [w581 w667]
                  disable-tunnel: w563 -> [w580 w666]
                  disable-tunnel: w562 -> [w579 _]
                  disable-tunnel: w561 -> [w578 _]
                  disable-tunnel: [w577 _] -> w560
                  disable-tunnel: [w576 _] -> w559
                  disable-tunnel: w558 -> [_ w664]
                  frame Disabled {
                    n201 = case shown="참" w580 {
                      tunnel: w581 -> [_ w590]
                      tunnel: ["No Decesion" ("메시지") w589] -> w575
                      tunnel: w579 -> [w582 w588]
                      tunnel: w578 -> [w583 w587]
                      tunnel: [w583 w586] -> w577
                      tunnel: [w582 w585] -> w576
                      frame False {
                      }
                      frame True {
                        n202 = disable-structure shown="Enabled" {
                          disable-tunnel: [w596 _ "" ("메시지")] -> w589
                          disable-tunnel: w590 -> [w595 w638 _]
                          disable-tunnel: w588 -> [w594 _ _]
                          disable-tunnel: w587 -> [w593 _ _]
                          disable-tunnel: [w592 _ _] -> w586
                          disable-tunnel: [w591 _ _] -> w585
                          frame Enabled {
                            n203 = case shown="1" w595 {
                              tunnel: ["전원" ("메시지") "음향 UP" ("메시지") "채널 UP" ("메시지") "전체종료" ("메시지") "음향 Down" ("메시지") "채널 Down" ("메시지") "No Decesion" ("메시지")] -> w596
                              tunnel: w594 -> [w600 w607 w613 w618 w624 w631 w635]
                              tunnel: w593 -> [w599 w606 w614 w619 w623 w630 w636]
                              tunnel: [w598 w605 w612 w619 w622 w629 w636] -> w592
                              tunnel: [w597 w604 w611 w618 w621 w628 w635] -> w591
                              frame 0 {
                                n204 = VISA Write(VISA resource name=w599, write buffer="0", error in (no error)=w600) -> (VISA resource name out=w598:refnum<visa-resource-name>, error out=w597:errorcluster)  [unwired: 1 out]
                                n205 = Wait (ms)(milliseconds to wait=u32 10) -> ()  [unwired: 1 out]
                              }
                              frame 1 {
                                n206 = VISA Write(VISA resource name=w606, write buffer="L", error in (no error)=w607) -> (VISA resource name out=w605:refnum<visa-resource-name>, error out=w604:errorcluster)  [unwired: 1 out]
                                n207 = Wait (ms)(milliseconds to wait=u32 10) -> ()  [unwired: 1 out]
                              }
                              frame 2 {
                                n208 = VISA Write(VISA resource name=w614, write buffer="J", error in (no error)=w613) -> (VISA resource name out=w612:refnum<visa-resource-name>, error out=w611:errorcluster)  [unwired: 1 out]
                                n209 = Wait (ms)(milliseconds to wait=u32 10) -> ()  [unwired: 1 out]
                              }
                              frame 3 {
                              }
                              frame 4 {
                                n210 = VISA Write(VISA resource name=w623, write buffer="M", error in (no error)=w624) -> (VISA resource name out=w622:refnum<visa-resource-name>, error out=w621:errorcluster)  [unwired: 1 out]
                                n211 = Wait (ms)(milliseconds to wait=u32 10) -> ()  [unwired: 1 out]
                              }
                              frame 5 {
                                n212 = VISA Write(VISA resource name=w630, write buffer="K", error in (no error)=w631) -> (VISA resource name out=w629:refnum<visa-resource-name>, error out=w628:errorcluster)  [unwired: 1 out]
                                n213 = Wait (ms)(milliseconds to wait=u32 10) -> ()  [unwired: 1 out]
                              }
                              frame 9, Default {
                              }
                            }
                          }
                          frame Disabled {
                            n214 = case shown="0, 기본" w638 {
                              frame 0, Default {
                                n215 = Current VI's Path() -> (path=w640:path)
                                n216 = Strip Path(path=w640) -> (stripped path=w641:path)  [unwired: 1 out]
                                n217 = Build Path(base path=w641, name or relative path="0.wav" ("이름 또는 상대 경로")) -> (appended path=w639:path)
                                n218 = call "Sound_Sub.vi"("path"=w639) -> ()
                              }
                              frame 2 {
                                n219 = Current VI's Path() -> (path=w643:path)
                                n220 = Strip Path(path=w643) -> (stripped path=w644:path)  [unwired: 1 out]
                                n221 = Build Path(base path=w644, name or relative path="2.wav" ("이름 또는 상대 경로")) -> (appended path=w646:path)
                                n222 = call "Sound_Sub.vi"("path"=w646) -> ()
                              }
                              frame 3 {
                                n223 = Current VI's Path() -> (path=w647:path)
                                n224 = Strip Path(path=w647) -> (stripped path=w648:path)  [unwired: 1 out]
                                n225 = Build Path(base path=w648, name or relative path="3.wav" ("이름 또는 상대 경로")) -> (appended path=w650:path)
                                n226 = call "Sound_Sub.vi"("path"=w650) -> ()
                              }
                              frame 4 {
                                n227 = Current VI's Path() -> (path=w651:path)
                                n228 = Strip Path(path=w651) -> (stripped path=w652:path)  [unwired: 1 out]
                                n229 = Build Path(base path=w652, name or relative path="4.wav" ("이름 또는 상대 경로")) -> (appended path=w654:path)
                                n230 = call "Sound_Sub.vi"("path"=w654) -> ()
                              }
                              frame 5 {
                                n231 = Current VI's Path() -> (path=w655:path)
                                n232 = Strip Path(path=w655) -> (stripped path=w656:path)  [unwired: 1 out]
                                n233 = Build Path(base path=w656, name or relative path="5.wav" ("이름 또는 상대 경로")) -> (appended path=w658:path)
                                n234 = call "Sound_Sub.vi"("path"=w658) -> ()
                              }
                              frame 1 {
                                n235 = Current VI's Path() -> (path=w660:path)
                                n236 = Strip Path(path=w660) -> (stripped path=w661:path)  [unwired: 1 out]
                                n237 = Build Path(base path=w661, name or relative path="1.wav" ("이름 또는 상대 경로")) -> (appended path=w659:path)
                                n238 = call "Sound_Sub.vi"("path"=w659) -> ()
                              }
                            }
                          }
                          frame Disabled {
                          }
                        }
                      }
                    }
                    n239 = global write "Control_Panel_정리.vi" "선택된 기능"(w575) -> ()
                  }
                  frame Enabled {
                    n240 = flat-sequence {
                      tunnel: w667 -> [w671]
                      tunnel: w666 -> [w670]
                      tunnel: [w668] -> w665
                      tunnel: w664 -> [w668]
                      tunnel: w665 -> [w710]
                      frame #0 {
                        n241 = case shown="참" w670 {
                          tunnel: w671 -> [_ w674]
                          tunnel: ["No Decesion" ("메시지") w673] -> w669
                          frame False {
                          }
                          frame True {
                            n242 = disable-structure shown="활성화" {
                              disable-tunnel: [w676 _ "" ("메시지")] -> w673
                              disable-tunnel: w674 -> [w675 w684 _]
                              frame Enabled {
                                n243 = case shown="4" w675 {
                                tunnel: ["온도" ("메시지") "자판" ("메시지") "침대" ("메시지") "용변" ("메시지") "기계" ("메시지") "응급" ("메시지") "No Decesion" ("메시지")] -> w676
                                frame 0 {
                                }
                                frame 1 {
                                }
                                frame 2 {
                                }
                                frame 3 {
                                }
                                frame 4 {
                                }
                                frame 5 {
                                }
                                frame 9, Default {
                                }
                                }
                              }
                              frame Disabled {
                                n244 = case shown="4" w684 {
                                frame 0, Default {
                                n245 = Current VI's Path() -> (path=w686:path)
                                n246 = Strip Path(path=w686) -> (stripped path=w687:path)  [unwired: 1 out]
                                n247 = Build Path(base path=w687, name or relative path="0.wav" ("이름 또는 상대 경로")) -> (appended path=w685:path)
                                n248 = call "Sound_Sub.vi"("path"=w685) -> ()
                                }
                                frame 2 {
                                n249 = Current VI's Path() -> (path=w689:path)
                                n250 = Strip Path(path=w689) -> (stripped path=w690:path)  [unwired: 1 out]
                                n251 = Build Path(base path=w690, name or relative path="2.wav" ("이름 또는 상대 경로")) -> (appended path=w692:path)
                                n252 = call "Sound_Sub.vi"("path"=w692) -> ()
                                }
                                frame 3 {
                                n253 = Current VI's Path() -> (path=w693:path)
                                n254 = Strip Path(path=w693) -> (stripped path=w694:path)  [unwired: 1 out]
                                n255 = Build Path(base path=w694, name or relative path="3.wav" ("이름 또는 상대 경로")) -> (appended path=w696:path)
                                n256 = call "Sound_Sub.vi"("path"=w696) -> ()
                                }
                                frame 4 {
                                n257 = Current VI's Path() -> (path=w697:path)
                                n258 = Strip Path(path=w697) -> (stripped path=w698:path)  [unwired: 1 out]
                                n259 = Build Path(base path=w698, name or relative path="4.wav" ("이름 또는 상대 경로")) -> (appended path=w700:path)
                                n260 = call "Sound_Sub.vi"("path"=w700) -> ()
                                }
                                frame 5 {
                                n261 = Current VI's Path() -> (path=w701:path)
                                n262 = Strip Path(path=w701) -> (stripped path=w702:path)  [unwired: 1 out]
                                n263 = Build Path(base path=w702, name or relative path="5.wav" ("이름 또는 상대 경로")) -> (appended path=w704:path)
                                n264 = call "Sound_Sub.vi"("path"=w704) -> ()
                                }
                                frame 1 {
                                n265 = Current VI's Path() -> (path=w706:path)
                                n266 = Strip Path(path=w706) -> (stripped path=w707:path)  [unwired: 1 out]
                                n267 = Build Path(base path=w707, name or relative path="1.wav" ("이름 또는 상대 경로")) -> (appended path=w705:path)
                                n268 = call "Sound_Sub.vi"("path"=w705) -> ()
                                }
                                }
                              }
                              frame Disabled {
                              }
                            }
                          }
                        }
                        n269 = global write "Control_Panel_정리.vi" "선택된 기능"(w669) -> ()
                      }
                      frame #1 {
                        n270 = case shown="참" w710 {
                          frame False {
                          }
                          frame True {
                            n271 = global read "Control_Panel_정리.vi" "Send_Interaction"() -> (w713:u8)
                            n272 = stacked-sequence {
                              tunnel: w713 -> [w715 _ w719]
                              tunnel: u32 0 ("dwFlags") -> [w714 _ w718]
                              frame #0 {
                                n273 = dll-call lib="User32.dll" fn="keybd_event"("bVk"=w715, "bScan"=w714, "dwFlags"=w714, "dwExtraInfo"=w714) -> ()  [unwired: 8 in, 2 out]
                              }
                              frame #1 {
                                n274 = Wait Until Next ms Multiple(millisecond multiple=u32 250) -> ()  [unwired: 1 out]
                              }
                              frame #2 {
                                n275 = dll-call lib="User32.dll" fn="keybd_event"("bVk"=w719, "bScan"=w718, "dwFlags"=u32 2, "dwExtraInfo"=w718) -> ()  [unwired: 8 in, 2 out]
                              }
                            }
                            n276 = global write "Control_Panel_정리.vi" "Switch"(FALSE ("Switch")) -> ()
                          }
                        }
                      }
                    }
                  }
                }
              }
            }
            n277 = global write "Control_Panel_정리.vi" "ERP_Pannel"(TRUE ("ERP_Pannel")) -> ()
            n278 = Build Array (concatenate)(w152, w151) -> (w145:dbl[])
            n279 = Increment(x=w141) -> (x+1=w140:i32)
          }
        }
        n280 = global read "Control_Panel_정리.vi" "정지"() -> (w95:bool)
      }
      n281 = global write "Control_Panel_정리.vi" "Acquisition Mode"(TRUE ("Device Control Enabled")) -> ()
      n282 = global write "Control_Panel_정리.vi" "Device Control Enabled"(FALSE ("Device Control Enabled")) -> ()
    }
    frame #3 {
      n283 = disable-structure shown="Disabled" {
        disable-tunnel: w722 -> [w766 _]
        disable-tunnel: w721 -> [w765 _]
        frame Disabled {
          n284 = VISA Close(VISA resource name=w766, error in (no error)=w765) -> ()  [unwired: 1 out]
        }
        frame Enabled {
        }
      }
      n285 = dll-call lib="C:/Users/Server/Desktop/NeuroSky/NeuroSky_Dll_Call/Debug/NeuroSky_Dll_Call.dll" fn="FreeConnection"() -> ()  [unwired: 4 in, 2 out]
      n286 = global write "Control_Panel_정리.vi" "Acquisition Mode"(FALSE ("Device Control Enabled")) -> ()
      n287 = global write "Control_Panel_정리.vi" "Communication Stopped"(TRUE ("Device Control Enabled")) -> ()
      n288 = Build Path(base path=w725, name or relative path="Brain.txt") -> (appended path=w764:path)
      n289 = Build Path(base path=w725, name or relative path="selectedtarget.txt") -> (appended path=w756:path)
      n290 = Build Path(base path=w725, name or relative path="mius_flash_order.txt") -> (appended path=w761:path)
      n291 = Build Path(base path=w725, name or relative path="Target_order.txt") -> (appended path=w751:path)
      n292 = Build Path(base path=w725, name or relative path="Accuracy.txt") -> (appended path=w754:path)
      n293 = Build Path(base path=w725, name or relative path="ERP_발생_total.txt") -> (appended path=w744:path)
      n294 = Build Path(base path=w725, name or relative path="ERP_all_icon.txt") -> (appended path=w740:path)
      n295 = Build Path(base path=w725, name or relative path="ERP_total.txt") -> (appended path=w728:path)
      n296 = Build Path(base path=w725, name or relative path="SWLDA_hyperplane_value.txt") -> (appended path=w736:path)
      n297 = Build Path(base path=w725, name or relative path="decision_value.txt") -> (appended path=w733:path)
      n298 = call-poly <vilib>:"Write To Spreadsheet File.vi"("format (%.3f)"="%.6f", "1D data"=w720, "file path (dialog if empty)"=w764) -> ()  [unwired: 5 in, 1 out]
      n299 = call-poly <vilib>:"Write To Spreadsheet File.vi"("1D data"=w755, "file path (dialog if empty)"=w756) -> ()  [unwired: 6 in, 1 out]
      n300 = call-poly <vilib>:"Write To Spreadsheet File.vi"("transpose? (no:F)"=TRUE, "2D data"=w759, "file path (dialog if empty)"=w761) -> ()  [unwired: 5 in, 1 out]
      n301 = call-poly <vilib>:"Write To Spreadsheet File.vi"("transpose? (no:F)"=TRUE, "1D data"=w748, "file path (dialog if empty)"=w751) -> ()  [unwired: 5 in, 1 out]
      n302 = call-poly <vilib>:"Write To Spreadsheet File.vi"("1D data"=w752, "file path (dialog if empty)"=w754) -> ()  [unwired: 6 in, 1 out]
      n303 = call-poly <vilib>:"Write To Spreadsheet File.vi"("transpose? (no:F)"=TRUE, "1D data"=w742, "file path (dialog if empty)"=w744) -> ()  [unwired: 5 in, 1 out]
      n304 = call-poly <vilib>:"Write To Spreadsheet File.vi"("transpose? (no:F)"=TRUE, "format (%.3f)"="%.6f", "2D data"=w737, "file path (dialog if empty)"=w740) -> ()  [unwired: 4 in, 1 out]
      n305 = call-poly <vilib>:"Write To Spreadsheet File.vi"("transpose? (no:F)"=TRUE, "format (%.3f)"="%.6f", "2D data"=w726, "file path (dialog if empty)"=w728) -> ()  [unwired: 4 in, 1 out]
      n306 = call-poly <vilib>:"Write To Spreadsheet File.vi"("format (%.3f)"="%.6f", "1D data"=w734, "file path (dialog if empty)"=w736) -> ()  [unwired: 5 in, 1 out]
      n307 = call-poly <vilib>:"Write To Spreadsheet File.vi"("format (%.3f)"="%.6f", "1D data"=w731, "file path (dialog if empty)"=w733) -> ()  [unwired: 5 in, 1 out]
    }
    frame #4 {
      n308 = global write "Control_Panel_정리.vi" "Communication Stopped"(FALSE ("Device Control Enabled")) -> ()
    }
  }
